vi "create.vi"(8 "error in (no error)":errorcluster, 10 "Default Goal Amount":dbl, 11 "Name":string) -> (0 "error out":errorcluster, 3 "Category out":refnum<class "Category.lvclass">)   [LabVIEW 2018, in "Category.lvclass"]
uses:
  Category.lvclass
  Category.lvclass/Category.ctl
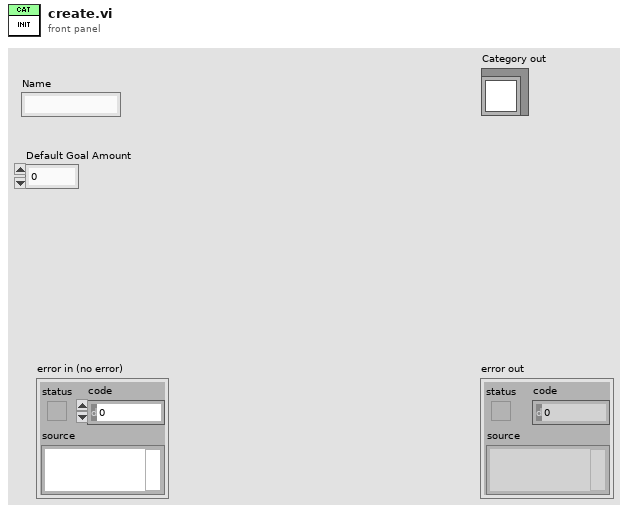
[diagram p1: front panel]
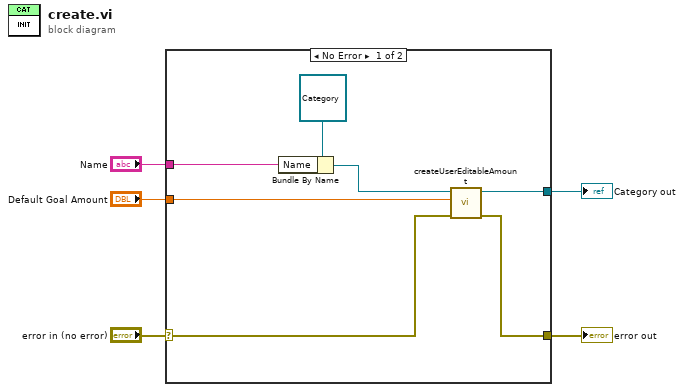
[diagram p0: block diagram]
diagram:
  n1 = case shown="No Error" "error in (no error)" {
    selector: "error in (no error)" -> [w11 w13]
    tunnel: [w6 w13] -> w4
    tunnel: [w7 _] -> w3
    tunnel: "Default Goal Amount" -> [w10 _]
    tunnel: "Name" -> [w12 _]
    frame No Error {
      n2 = Bundle By Name(cluster=refnum<class "Category.lvclass"> refnum ("Category.lvclass"), "Name"=w12) -> (w8:refnum<class "Category.lvclass">)
      n3 = call-dynamic "createUserEditableAmount.vi"("error in (no error)"=w11, "Create"=w10, "UserEditableAmount"=w8) -> ("error out"=w6:errorcluster, "UserEditableAmount out"=w7:refnum<class "Category.lvclass">)  [unwired: 7 in]
    }
    frame Error {
    }
  }
  "error out" <- w4
  "Category out" <- w3
